vi "Read Attributes.vi"(11 "Response Msg":refnum<class "Response Msg.lvclass">) -> (2 "Payload":cluster{"Response":string})   [LabVIEW 2019, in "Serial.lvlib" / "Response Msg.lvclass"]
uses:
  Response Msg.lvclass
  Response Msg.lvclass/Response Msg.ctl
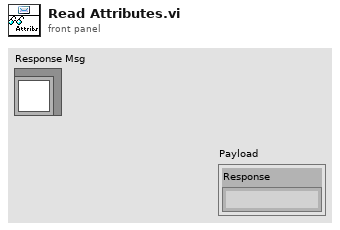
[diagram p1: front panel]
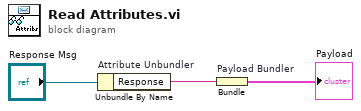
[diagram p0: block diagram]
diagram:
  n1 = Unbundle By Name "Attribute Unbundler"("Response Msg") -> ("Response"=w1:string)
  n2 = Bundle "Payload Bundler"("Response"=w1) -> (→"Payload":cluster{"Response":string})  [unwired: 1 in]
